vi "Main_RT Feedback.vi"() -> ()   [LabVIEW 2010]
uses:
  <vilib>/Analysis/Matrix/Datatypes/RealMatrix.ctl
  <vilib>/Utility/miscctls.llb/LV3DPointTypeDef.ctl
  <vilib>/Utility/miscctls.llb/LVRectTypeDef.ctl
  <vilib>/picture/3D Picture Control/NI_3D Picture Control.lvlib
  <vilib>/Analysis/Matrix/NI_Matrix.lvlib
panel:
  out "Number of Markers\nfor first BodyDef":i32
  in  "STOP":bool
  out "Unnamed Data":sgl[](array[numeric])
  out "nUnidentifiedMarkers":i32
  out "Unidentified Markers Ptr":u32
  out "Marker Data":sgl[][](array[numeric])
  out "Marker Names\nfor first BodyDef":string[](array[string])
  out "szMarkerNames":u32[](array[numeric])
  out "nMarkers":i32[](array[numeric])
  in  "sBodyDefs":T1
  out "iFrame 2":i32
  in  "Host IP":string="10.1.1.200"
  in  "Local IP":string="10.1.1.150"
  in  "DLL Path":path=path "C:/Program Files (x86)/Motion Analysis/SDK2/Cortex_SDK.dll"
  in  "Write Data to TRC?":bool=TRUE
  out "Arm Refs":T2
  out "3D Picture":refnum<vi>
  in  "Shoulder":bool=TRUE
  out "SceneWindow":refnum<vi>
  # "RealTime Feedback Program for Tracking Shoulder Motion"
  # "Left"
  # "Right"
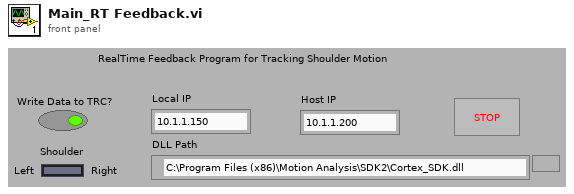
[diagram p1: front panel]
types:
  T1 = cluster{"nBodyDefs":i32, "sBodyDef":cluster{"szName":u32, "nMarkers":i32, "szMarkerNames":u32, "sHierarchy":cluster{"nSegments":i32, "szSegmentNames":u32, "iParents":u32}, "nDofs":i32, "szDefNames":u32}, "nAnalogChannels":i32, "szAnalogChannelNames":u32, "nForcePlates":i32, "AllocatedSpace":u32}
  T2 = cluster{"R Arm":refnum<vi>, "L Arm":refnum<vi>, "R SJC":refnum<vi>, "L EJC":refnum<vi>, "R EJC":refnum<vi>}
  T3 = typedef "NI_Matrix.lvlib/RealMatrix.ctl" = dbl[][]
  T4 = enum16{"Open", "Minimized", "Maximized", "Hidden"}
  T5 = typedef "LV3DPointTypeDef.ctl" = cluster{"X":sgl, "Y":sgl, "Z":sgl}
  T6 = typedef "LVRectTypeDef.ctl" = cluster{"Left":i16, "Top":i16, "Right":i16, "Bottom":i16}
  T7 = cluster{"Shoulder Axis[0]":dbl, "Shoulder Axis[1]":dbl, "Shoulder Axis[2]":dbl}
  T8 = cluster{dbl, "Shoulder Axis":cluster{"Shoulder Axis[0]":dbl, "Shoulder Axis[1]":dbl, "Shoulder Axis[2]":dbl}, dbl, "Shoulder Axis":cluster{"Shoulder Axis[0]":dbl, "Shoulder Axis[1]":dbl, "Shoulder Axis[2]":dbl}, "Humerus Coord Sys":T3, "Shoulder Axis":cluster{"Shoulder Axis[0]":dbl, "Shoulder Axis[1]":dbl, "Shoulder Axis[2]":dbl}}
  T9 = cluster{"szName":u32, "nMarkers":i32, "szMarkerNames":u32, "sHierarchy":cluster{"nSegments":i32, "szSegmentNames":u32, "iParents":u32}, "nDofs":i32, "szDefNames":u32}
  T10 = cluster{"[0]":cluster{"szName":u32, "nMarkers":i32, "szMarkerNames":u32, "sHierarchy":cluster{"nSegments":i32, "szSegmentNames":u32, "iParents":u32}, "nDofs":i32, "szDefNames":u32}, "[1]":cluster{"szName":u32, "nMarkers":i32, "szMarkerNames":u32, "sHierarchy":cluster{"nSegments":i32, "szSegmentNames":u32, "iParents":u32}, "nDofs":i32, "szDefNames":u32}, "[2]":cluster{"szName":u32, "nMarkers":i32, "szMarkerNames":u32, "sHierarchy":cluster{"nSegments":i32, "szSegmentNames":u32, "iParents":u32}, "nDofs":i32, "szDefNames":u32}, "[3]":cluster{"szName":u32, "nMarkers":i32, "szMarkerNames":u32, "sHierarchy":cluster{"nSegments":i32, "szSegmentNames":u32, "iParents":u32}, "nDofs":i32, "szDefNames":u32}, "[4]":cluster{"szName":u32, "nMarkers":i32, "szMarkerNames":u32, "sHierarchy":cluster{"nSegments":i32, "szSegmentNames":u32, "iParents":u32}, "nDofs":i32, "szDefNames":u32}, "[5]":cluster{"szName":u32, "nMarkers":i32, "szMarkerNames":u32, "sHierarchy":cluster{"nSegments":i32, "szSegmentNames":u32, "iParents":u32}, "nDofs":i32, "szDefNames":u32}, "[6]":cluster{"szName":u32, "nMarkers":i32, "szMarkerNames":u32, "sHierarchy":cluster{"nSegments":i32, "szSegmentNames":u32, "iParents":u32}, "nDofs":i32, "szDefNames":u32}, "[7]":cluster{"szName":u32, "nMarkers":i32, "szMarkerNames":u32, "sHierarchy":cluster{"nSegments":i32, "szSegmentNames":u32, "iParents":u32}, "nDofs":i32, "szDefNames":u32}, "[8]":cluster{"szName":u32, "nMarkers":i32, "szMarkerNames":u32, "sHierarchy":cluster{"nSegments":i32, "szSegmentNames":u32, "iParents":u32}, "nDofs":i32, "szDefNames":u32}, "[9]":cluster{"szName":u32, "nMarkers":i32, "szMarkerNames":u32, "sHierarchy":cluster{"nSegments":i32, "szSegmentNames":u32, "iParents":u32}, "nDofs":i32, "szDefNames":u32}, "[10]":cluster{"szName":u32, "nMarkers":i32, "szMarkerNames":u32, "sHierarchy":cluster{"nSegments":i32, "szSegmentNames":u32, "iParents":u32}, "nDofs":i32, "szDefNames":u32}, "[11]":cluster{"szName":u32, "nMarkers":i32, "szMarkerNames":u32, "sHierarchy":cluster{"nSegments":i32, "szSegmentNames":u32, "iParents":u32}, "nDofs":i32, "szDefNames":u32}, "[12]":cluster{"szName":u32, "nMarkers":i32, "szMarkerNames":u32, "sHierarchy":cluster{"nSegments":i32, "szSegmentNames":u32, "iParents":u32}, "nDofs":i32, "szDefNames":u32}, "[13]":cluster{"szName":u32, "nMarkers":i32, "szMarkerNames":u32, "sHierarchy":cluster{"nSegments":i32, "szSegmentNames":u32, "iParents":u32}, "nDofs":i32, "szDefNames":u32}, "[14]":cluster{"szName":u32, "nMarkers":i32, "szMarkerNames":u32, "sHierarchy":cluster{"nSegments":i32, "szSegmentNames":u32, "iParents":u32}, "nDofs":i32, "szDefNames":u32}, "[15]":cluster{"szName":u32, "nMarkers":i32, "szMarkerNames":u32, "sHierarchy":cluster{"nSegments":i32, "szSegmentNames":u32, "iParents":u32}, "nDofs":i32, "szDefNames":u32}, "[16]":cluster{"szName":u32, "nMarkers":i32, "szMarkerNames":u32, "sHierarchy":cluster{"nSegments":i32, "szSegmentNames":u32, "iParents":u32}, "nDofs":i32, "szDefNames":u32}, "[17]":cluster{"szName":u32, "nMarkers":i32, "szMarkerNames":u32, "sHierarchy":cluster{"nSegments":i32, "szSegmentNames":u32, "iParents":u32}, "nDofs":i32, "szDefNames":u32}, "[18]":cluster{"szName":u32, "nMarkers":i32, "szMarkerNames":u32, "sHierarchy":cluster{"nSegments":i32, "szSegmentNames":u32, "iParents":u32}, "nDofs":i32, "szDefNames":u32}, "[19]":cluster{"szName":u32, "nMarkers":i32, "szMarkerNames":u32, "sHierarchy":cluster{"nSegments":i32, "szSegmentNames":u32, "iParents":u32}, "nDofs":i32, "szDefNames":u32}, "[20]":cluster{"szName":u32, "nMarkers":i32, "szMarkerNames":u32, "sHierarchy":cluster{"nSegments":i32, "szSegmentNames":u32, "iParents":u32}, "nDofs":i32, "szDefNames":u32}, "[21]":cluster{"szName":u32, "nMarkers":i32, "szMarkerNames":u32, "sHierarchy":cluster{"nSegments":i32, "szSegmentNames":u32, "iParents":u32}, "nDofs":i32, "szDefNames":u32}, "[22]":cluster{"szName":u32, "nMarkers":i32, "szMarkerNames":u32, "sHierarchy":cluster{"nSegments":i32, "szSegmentNames":u32, "iParents":u32}, "nDofs":i32, "szDefNames":u32}, "[23]":cluster{"szName":u32, "nMarkers":i32, "szMarkerNames":u32, "sHierarchy":cluster{"nSegments":i32, "szSegmentNames":u32, "iParents":u32}, "nDofs":i32, "szDefNames":u32}, "[24]":cluster{"szName":u32, "nMarkers":i32, "szMarkerNames":u32, "sHierarchy":cluster{"nSegments":i32, "szSegmentNames":u32, "iParents":u32}, "nDofs":i32, "szDefNames":u32}, "[25]":cluster{"szName":u32, "nMarkers":i32, "szMarkerNames":u32, "sHierarchy":cluster{"nSegments":i32, "szSegmentNames":u32, "iParents":u32}, "nDofs":i32, "szDefNames":u32}, "[26]":cluster{"szName":u32, "nMarkers":i32, "szMarkerNames":u32, "sHierarchy":cluster{"nSegments":i32, "szSegmentNames":u32, "iParents":u32}, "nDofs":i32, "szDefNames":u32}, "[27]":cluster{"szName":u32, "nMarkers":i32, "szMarkerNames":u32, "sHierarchy":cluster{"nSegments":i32, "szSegmentNames":u32, "iParents":u32}, "nDofs":i32, "szDefNames":u32}, "[28]":cluster{"szName":u32, "nMarkers":i32, "szMarkerNames":u32, "sHierarchy":cluster{"nSegments":i32, "szSegmentNames":u32, "iParents":u32}, "nDofs":i32, "szDefNames":u32}, "[29]":cluster{"szName":u32, "nMarkers":i32, "szMarkerNames":u32, "sHierarchy":cluster{"nSegments":i32, "szSegmentNames":u32, "iParents":u32}, "nDofs":i32, "szDefNames":u32}, "[30]":cluster{"szName":u32, "nMarkers":i32, "szMarkerNames":u32, "sHierarchy":cluster{"nSegments":i32, "szSegmentNames":u32, "iParents":u32}, "nDofs":i32, "szDefNames":u32}, "[31]":cluster{"szName":u32, "nMarkers":i32, "szMarkerNames":u32, "sHierarchy":cluster{"nSegments":i32, "szSegmentNames":u32, "iParents":u32}, "nDofs":i32, "szDefNames":u32}, "[32]":cluster{"szName":u32, "nMarkers":i32, "szMarkerNames":u32, "sHierarchy":cluster{"nSegments":i32, "szSegmentNames":u32, "iParents":u32}, "nDofs":i32, "szDefNames":u32}, "[33]":cluster{"szName":u32, "nMarkers":i32, "szMarkerNames":u32, "sHierarchy":cluster{"nSegments":i32, "szSegmentNames":u32, "iParents":u32}, "nDofs":i32, "szDefNames":u32}, "[34]":cluster{"szName":u32, "nMarkers":i32, "szMarkerNames":u32, "sHierarchy":cluster{"nSegments":i32, "szSegmentNames":u32, "iParents":u32}, "nDofs":i32, "szDefNames":u32}, "[35]":cluster{"szName":u32, "nMarkers":i32, "szMarkerNames":u32, "sHierarchy":cluster{"nSegments":i32, "szSegmentNames":u32, "iParents":u32}, "nDofs":i32, "szDefNames":u32}, "[36]":cluster{"szName":u32, "nMarkers":i32, "szMarkerNames":u32, "sHierarchy":cluster{"nSegments":i32, "szSegmentNames":u32, "iParents":u32}, "nDofs":i32, "szDefNames":u32}, "[37]":cluster{"szName":u32, "nMarkers":i32, "szMarkerNames":u32, "sHierarchy":cluster{"nSegments":i32, "szSegmentNames":u32, "iParents":u32}, "nDofs":i32, "szDefNames":u32}, "[38]":cluster{"szName":u32, "nMarkers":i32, "szMarkerNames":u32, "sHierarchy":cluster{"nSegments":i32, "szSegmentNames":u32, "iParents":u32}, "nDofs":i32, "szDefNames":u32}, "[39]":cluster{"szName":u32, "nMarkers":i32, "szMarkerNames":u32, "sHierarchy":cluster{"nSegments":i32, "szSegmentNames":u32, "iParents":u32}, "nDofs":i32, "szDefNames":u32}, "[40]":cluster{"szName":u32, "nMarkers":i32, "szMarkerNames":u32, "sHierarchy":cluster{"nSegments":i32, "szSegmentNames":u32, "iParents":u32}, "nDofs":i32, "szDefNames":u32}, "[41]":cluster{"szName":u32, "nMarkers":i32, "szMarkerNames":u32, "sHierarchy":cluster{"nSegments":i32, "szSegmentNames":u32, "iParents":u32}, "nDofs":i32, "szDefNames":u32}, "[42]":cluster{"szName":u32, "nMarkers":i32, "szMarkerNames":u32, "sHierarchy":cluster{"nSegments":i32, "szSegmentNames":u32, "iParents":u32}, "nDofs":i32, "szDefNames":u32}, "[43]":cluster{"szName":u32, "nMarkers":i32, "szMarkerNames":u32, "sHierarchy":cluster{"nSegments":i32, "szSegmentNames":u32, "iParents":u32}, "nDofs":i32, "szDefNames":u32}, "[44]":cluster{"szName":u32, "nMarkers":i32, "szMarkerNames":u32, "sHierarchy":cluster{"nSegments":i32, "szSegmentNames":u32, "iParents":u32}, "nDofs":i32, "szDefNames":u32}, "[45]":cluster{"szName":u32, "nMarkers":i32, "szMarkerNames":u32, "sHierarchy":cluster{"nSegments":i32, "szSegmentNames":u32, "iParents":u32}, "nDofs":i32, "szDefNames":u32}, "[46]":cluster{"szName":u32, "nMarkers":i32, "szMarkerNames":u32, "sHierarchy":cluster{"nSegments":i32, "szSegmentNames":u32, "iParents":u32}, "nDofs":i32, "szDefNames":u32}, "[47]":cluster{"szName":u32, "nMarkers":i32, "szMarkerNames":u32, "sHierarchy":cluster{"nSegments":i32, "szSegmentNames":u32, "iParents":u32}, "nDofs":i32, "szDefNames":u32}, "[48]":cluster{"szName":u32, "nMarkers":i32, "szMarkerNames":u32, "sHierarchy":cluster{"nSegments":i32, "szSegmentNames":u32, "iParents":u32}, "nDofs":i32, "szDefNames":u32}, "[49]":cluster{"szName":u32, "nMarkers":i32, "szMarkerNames":u32, "sHierarchy":cluster{"nSegments":i32, "szSegmentNames":u32, "iParents":u32}, "nDofs":i32, "szDefNames":u32}, "[50]":cluster{"szName":u32, "nMarkers":i32, "szMarkerNames":u32, "sHierarchy":cluster{"nSegments":i32, "szSegmentNames":u32, "iParents":u32}, "nDofs":i32, "szDefNames":u32}, "[51]":cluster{"szName":u32, "nMarkers":i32, "szMarkerNames":u32, "sHierarchy":cluster{"nSegments":i32, "szSegmentNames":u32, "iParents":u32}, "nDofs":i32, "szDefNames":u32}, "[52]":cluster{"szName":u32, "nMarkers":i32, "szMarkerNames":u32, "sHierarchy":cluster{"nSegments":i32, "szSegmentNames":u32, "iParents":u32}, "nDofs":i32, "szDefNames":u32}, "[53]":cluster{"szName":u32, "nMarkers":i32, "szMarkerNames":u32, "sHierarchy":cluster{"nSegments":i32, "szSegmentNames":u32, "iParents":u32}, "nDofs":i32, "szDefNames":u32}, "[54]":cluster{"szName":u32, "nMarkers":i32, "szMarkerNames":u32, "sHierarchy":cluster{"nSegments":i32, "szSegmentNames":u32, "iParents":u32}, "nDofs":i32, "szDefNames":u32}, "[55]":cluster{"szName":u32, "nMarkers":i32, "szMarkerNames":u32, "sHierarchy":cluster{"nSegments":i32, "szSegmentNames":u32, "iParents":u32}, "nDofs":i32, "szDefNames":u32}, "[56]":cluster{"szName":u32, "nMarkers":i32, "szMarkerNames":u32, "sHierarchy":cluster{"nSegments":i32, "szSegmentNames":u32, "iParents":u32}, "nDofs":i32, "szDefNames":u32}, "[57]":cluster{"szName":u32, "nMarkers":i32, "szMarkerNames":u32, "sHierarchy":cluster{"nSegments":i32, "szSegmentNames":u32, "iParents":u32}, "nDofs":i32, "szDefNames":u32}, "[58]":cluster{"szName":u32, "nMarkers":i32, "szMarkerNames":u32, "sHierarchy":cluster{"nSegments":i32, "szSegmentNames":u32, "iParents":u32}, "nDofs":i32, "szDefNames":u32}, "[59]":cluster{"szName":u32, "nMarkers":i32, "szMarkerNames":u32, "sHierarchy":cluster{"nSegments":i32, "szSegmentNames":u32, "iParents":u32}, "nDofs":i32, "szDefNames":u32}, "[60]":cluster{"szName":u32, "nMarkers":i32, "szMarkerNames":u32, "sHierarchy":cluster{"nSegments":i32, "szSegmentNames":u32, "iParents":u32}, "nDofs":i32, "szDefNames":u32}, "[61]":cluster{"szName":u32, "nMarkers":i32, "szMarkerNames":u32, "sHierarchy":cluster{"nSegments":i32, "szSegmentNames":u32, "iParents":u32}, "nDofs":i32, "szDefNames":u32}, "[62]":cluster{"szName":u32, "nMarkers":i32, "szMarkerNames":u32, "sHierarchy":cluster{"nSegments":i32, "szSegmentNames":u32, "iParents":u32}, "nDofs":i32, "szDefNames":u32}, "[63]":cluster{"szName":u32, "nMarkers":i32, "szMarkerNames":u32, "sHierarchy":cluster{"nSegments":i32, "szSegmentNames":u32, "iParents":u32}, "nDofs":i32, "szDefNames":u32}, "[64]":cluster{"szName":u32, "nMarkers":i32, "szMarkerNames":u32, "sHierarchy":cluster{"nSegments":i32, "szSegmentNames":u32, "iParents":u32}, "nDofs":i32, "szDefNames":u32}, "[65]":cluster{"szName":u32, "nMarkers":i32, "szMarkerNames":u32, "sHierarchy":cluster{"nSegments":i32, "szSegmentNames":u32, "iParents":u32}, "nDofs":i32, "szDefNames":u32}, "[66]":cluster{"szName":u32, "nMarkers":i32, "szMarkerNames":u32, "sHierarchy":cluster{"nSegments":i32, "szSegmentNames":u32, "iParents":u32}, "nDofs":i32, "szDefNames":u32}, "[67]":cluster{"szName":u32, "nMarkers":i32, "szMarkerNames":u32, "sHierarchy":cluster{"nSegments":i32, "szSegmentNames":u32, "iParents":u32}, "nDofs":i32, "szDefNames":u32}, "[68]":cluster{"szName":u32, "nMarkers":i32, "szMarkerNames":u32, "sHierarchy":cluster{"nSegments":i32, "szSegmentNames":u32, "iParents":u32}, "nDofs":i32, "szDefNames":u32}, "[69]":cluster{"szName":u32, "nMarkers":i32, "szMarkerNames":u32, "sHierarchy":cluster{"nSegments":i32, "szSegmentNames":u32, "iParents":u32}, "nDofs":i32, "szDefNames":u32}, "[70]":cluster{"szName":u32, "nMarkers":i32, "szMarkerNames":u32, "sHierarchy":cluster{"nSegments":i32, "szSegmentNames":u32, "iParents":u32}, "nDofs":i32, "szDefNames":u32}, "[71]":cluster{"szName":u32, "nMarkers":i32, "szMarkerNames":u32, "sHierarchy":cluster{"nSegments":i32, "szSegmentNames":u32, "iParents":u32}, "nDofs":i32, "szDefNames":u32}, "[72]":cluster{"szName":u32, "nMarkers":i32, "szMarkerNames":u32, "sHierarchy":cluster{"nSegments":i32, "szSegmentNames":u32, "iParents":u32}, "nDofs":i32, "szDefNames":u32}, "[73]":cluster{"szName":u32, "nMarkers":i32, "szMarkerNames":u32, "sHierarchy":cluster{"nSegments":i32, "szSegmentNames":u32, "iParents":u32}, "nDofs":i32, "szDefNames":u32}, "[74]":cluster{"szName":u32, "nMarkers":i32, "szMarkerNames":u32, "sHierarchy":cluster{"nSegments":i32, "szSegmentNames":u32, "iParents":u32}, "nDofs":i32, "szDefNames":u32}, "[75]":cluster{"szName":u32, "nMarkers":i32, "szMarkerNames":u32, "sHierarchy":cluster{"nSegments":i32, "szSegmentNames":u32, "iParents":u32}, "nDofs":i32, "szDefNames":u32}, "[76]":cluster{"szName":u32, "nMarkers":i32, "szMarkerNames":u32, "sHierarchy":cluster{"nSegments":i32, "szSegmentNames":u32, "iParents":u32}, "nDofs":i32, "szDefNames":u32}, "[77]":cluster{"szName":u32, "nMarkers":i32, "szMarkerNames":u32, "sHierarchy":cluster{"nSegments":i32, "szSegmentNames":u32, "iParents":u32}, "nDofs":i32, "szDefNames":u32}, "[78]":cluster{"szName":u32, "nMarkers":i32, "szMarkerNames":u32, "sHierarchy":cluster{"nSegments":i32, "szSegmentNames":u32, "iParents":u32}, "nDofs":i32, "szDefNames":u32}, "[79]":cluster{"szName":u32, "nMarkers":i32, "szMarkerNames":u32, "sHierarchy":cluster{"nSegments":i32, "szSegmentNames":u32, "iParents":u32}, "nDofs":i32, "szDefNames":u32}, "[80]":cluster{"szName":u32, "nMarkers":i32, "szMarkerNames":u32, "sHierarchy":cluster{"nSegments":i32, "szSegmentNames":u32, "iParents":u32}, "nDofs":i32, "szDefNames":u32}, "[81]":cluster{"szName":u32, "nMarkers":i32, "szMarkerNames":u32, "sHierarchy":cluster{"nSegments":i32, "szSegmentNames":u32, "iParents":u32}, "nDofs":i32, "szDefNames":u32}, "[82]":cluster{"szName":u32, "nMarkers":i32, "szMarkerNames":u32, "sHierarchy":cluster{"nSegments":i32, "szSegmentNames":u32, "iParents":u32}, "nDofs":i32, "szDefNames":u32}, "[83]":cluster{"szName":u32, "nMarkers":i32, "szMarkerNames":u32, "sHierarchy":cluster{"nSegments":i32, "szSegmentNames":u32, "iParents":u32}, "nDofs":i32, "szDefNames":u32}, "[84]":cluster{"szName":u32, "nMarkers":i32, "szMarkerNames":u32, "sHierarchy":cluster{"nSegments":i32, "szSegmentNames":u32, "iParents":u32}, "nDofs":i32, "szDefNames":u32}, "[85]":cluster{"szName":u32, "nMarkers":i32, "szMarkerNames":u32, "sHierarchy":cluster{"nSegments":i32, "szSegmentNames":u32, "iParents":u32}, "nDofs":i32, "szDefNames":u32}, "[86]":cluster{"szName":u32, "nMarkers":i32, "szMarkerNames":u32, "sHierarchy":cluster{"nSegments":i32, "szSegmentNames":u32, "iParents":u32}, "nDofs":i32, "szDefNames":u32}, "[87]":cluster{"szName":u32, "nMarkers":i32, "szMarkerNames":u32, "sHierarchy":cluster{"nSegments":i32, "szSegmentNames":u32, "iParents":u32}, "nDofs":i32, "szDefNames":u32}, "[88]":cluster{"szName":u32, "nMarkers":i32, "szMarkerNames":u32, "sHierarchy":cluster{"nSegments":i32, "szSegmentNames":u32, "iParents":u32}, "nDofs":i32, "szDefNames":u32}, "[89]":cluster{"szName":u32, "nMarkers":i32, "szMarkerNames":u32, "sHierarchy":cluster{"nSegments":i32, "szSegmentNames":u32, "iParents":u32}, "nDofs":i32, "szDefNames":u32}, "[90]":cluster{"szName":u32, "nMarkers":i32, "szMarkerNames":u32, "sHierarchy":cluster{"nSegments":i32, "szSegmentNames":u32, "iParents":u32}, "nDofs":i32, "szDefNames":u32}, "[91]":cluster{"szName":u32, "nMarkers":i32, "szMarkerNames":u32, "sHierarchy":cluster{"nSegments":i32, "szSegmentNames":u32, "iParents":u32}, "nDofs":i32, "szDefNames":u32}, "[92]":cluster{"szName":u32, "nMarkers":i32, "szMarkerNames":u32, "sHierarchy":cluster{"nSegments":i32, "szSegmentNames":u32, "iParents":u32}, "nDofs":i32, "szDefNames":u32}, "[93]":cluster{"szName":u32, "nMarkers":i32, "szMarkerNames":u32, "sHierarchy":cluster{"nSegments":i32, "szSegmentNames":u32, "iParents":u32}, "nDofs":i32, "szDefNames":u32}, "[94]":cluster{"szName":u32, "nMarkers":i32, "szMarkerNames":u32, "sHierarchy":cluster{"nSegments":i32, "szSegmentNames":u32, "iParents":u32}, "nDofs":i32, "szDefNames":u32}, "[95]":cluster{"szName":u32, "nMarkers":i32, "szMarkerNames":u32, "sHierarchy":cluster{"nSegments":i32, "szSegmentNames":u32, "iParents":u32}, "nDofs":i32, "szDefNames":u32}, "[96]":cluster{"szName":u32, "nMarkers":i32, "szMarkerNames":u32, "sHierarchy":cluster{"nSegments":i32, "szSegmentNames":u32, "iParents":u32}, "nDofs":i32, "szDefNames":u32}, "[97]":cluster{"szName":u32, "nMarkers":i32, "szMarkerNames":u32, "sHierarchy":cluster{"nSegments":i32, "szSegmentNames":u32, "iParents":u32}, "nDofs":i32, "szDefNames":u32}, "[98]":cluster{"szName":u32, "nMarkers":i32, "szMarkerNames":u32, "sHierarchy":cluster{"nSegments":i32, "szSegmentNames":u32, "iParents":u32}, "nDofs":i32, "szDefNames":u32}, "[99]":cluster{"szName":u32, "nMarkers":i32, "szMarkerNames":u32, "sHierarchy":cluster{"nSegments":i32, "szSegmentNames":u32, "iParents":u32}, "nDofs":i32, "szDefNames":u32}}
  T11 = cluster{"nBodyDefs":i32, cluster{"[0]":cluster{"szName":u32, "nMarkers":i32, "szMarkerNames":u32, "sHierarchy":cluster{"nSegments":i32, "szSegmentNames":u32, "iParents":u32}, "nDofs":i32, "szDefNames":u32}, "[1]":cluster{"szName":u32, "nMarkers":i32, "szMarkerNames":u32, "sHierarchy":cluster{"nSegments":i32, "szSegmentNames":u32, "iParents":u32}, "nDofs":i32, "szDefNames":u32}, "[2]":cluster{"szName":u32, "nMarkers":i32, "szMarkerNames":u32, "sHierarchy":cluster{"nSegments":i32, "szSegmentNames":u32, "iParents":u32}, "nDofs":i32, "szDefNames":u32}, "[3]":cluster{"szName":u32, "nMarkers":i32, "szMarkerNames":u32, "sHierarchy":cluster{"nSegments":i32, "szSegmentNames":u32, "iParents":u32}, "nDofs":i32, "szDefNames":u32}, "[4]":cluster{"szName":u32, "nMarkers":i32, "szMarkerNames":u32, "sHierarchy":cluster{"nSegments":i32, "szSegmentNames":u32, "iParents":u32}, "nDofs":i32, "szDefNames":u32}, "[5]":cluster{"szName":u32, "nMarkers":i32, "szMarkerNames":u32, "sHierarchy":cluster{"nSegments":i32, "szSegmentNames":u32, "iParents":u32}, "nDofs":i32, "szDefNames":u32}, "[6]":cluster{"szName":u32, "nMarkers":i32, "szMarkerNames":u32, "sHierarchy":cluster{"nSegments":i32, "szSegmentNames":u32, "iParents":u32}, "nDofs":i32, "szDefNames":u32}, "[7]":cluster{"szName":u32, "nMarkers":i32, "szMarkerNames":u32, "sHierarchy":cluster{"nSegments":i32, "szSegmentNames":u32, "iParents":u32}, "nDofs":i32, "szDefNames":u32}, "[8]":cluster{"szName":u32, "nMarkers":i32, "szMarkerNames":u32, "sHierarchy":cluster{"nSegments":i32, "szSegmentNames":u32, "iParents":u32}, "nDofs":i32, "szDefNames":u32}, "[9]":cluster{"szName":u32, "nMarkers":i32, "szMarkerNames":u32, "sHierarchy":cluster{"nSegments":i32, "szSegmentNames":u32, "iParents":u32}, "nDofs":i32, "szDefNames":u32}, "[10]":cluster{"szName":u32, "nMarkers":i32, "szMarkerNames":u32, "sHierarchy":cluster{"nSegments":i32, "szSegmentNames":u32, "iParents":u32}, "nDofs":i32, "szDefNames":u32}, "[11]":cluster{"szName":u32, "nMarkers":i32, "szMarkerNames":u32, "sHierarchy":cluster{"nSegments":i32, "szSegmentNames":u32, "iParents":u32}, "nDofs":i32, "szDefNames":u32}, "[12]":cluster{"szName":u32, "nMarkers":i32, "szMarkerNames":u32, "sHierarchy":cluster{"nSegments":i32, "szSegmentNames":u32, "iParents":u32}, "nDofs":i32, "szDefNames":u32}, "[13]":cluster{"szName":u32, "nMarkers":i32, "szMarkerNames":u32, "sHierarchy":cluster{"nSegments":i32, "szSegmentNames":u32, "iParents":u32}, "nDofs":i32, "szDefNames":u32}, "[14]":cluster{"szName":u32, "nMarkers":i32, "szMarkerNames":u32, "sHierarchy":cluster{"nSegments":i32, "szSegmentNames":u32, "iParents":u32}, "nDofs":i32, "szDefNames":u32}, "[15]":cluster{"szName":u32, "nMarkers":i32, "szMarkerNames":u32, "sHierarchy":cluster{"nSegments":i32, "szSegmentNames":u32, "iParents":u32}, "nDofs":i32, "szDefNames":u32}, "[16]":cluster{"szName":u32, "nMarkers":i32, "szMarkerNames":u32, "sHierarchy":cluster{"nSegments":i32, "szSegmentNames":u32, "iParents":u32}, "nDofs":i32, "szDefNames":u32}, "[17]":cluster{"szName":u32, "nMarkers":i32, "szMarkerNames":u32, "sHierarchy":cluster{"nSegments":i32, "szSegmentNames":u32, "iParents":u32}, "nDofs":i32, "szDefNames":u32}, "[18]":cluster{"szName":u32, "nMarkers":i32, "szMarkerNames":u32, "sHierarchy":cluster{"nSegments":i32, "szSegmentNames":u32, "iParents":u32}, "nDofs":i32, "szDefNames":u32}, "[19]":cluster{"szName":u32, "nMarkers":i32, "szMarkerNames":u32, "sHierarchy":cluster{"nSegments":i32, "szSegmentNames":u32, "iParents":u32}, "nDofs":i32, "szDefNames":u32}, "[20]":cluster{"szName":u32, "nMarkers":i32, "szMarkerNames":u32, "sHierarchy":cluster{"nSegments":i32, "szSegmentNames":u32, "iParents":u32}, "nDofs":i32, "szDefNames":u32}, "[21]":cluster{"szName":u32, "nMarkers":i32, "szMarkerNames":u32, "sHierarchy":cluster{"nSegments":i32, "szSegmentNames":u32, "iParents":u32}, "nDofs":i32, "szDefNames":u32}, "[22]":cluster{"szName":u32, "nMarkers":i32, "szMarkerNames":u32, "sHierarchy":cluster{"nSegments":i32, "szSegmentNames":u32, "iParents":u32}, "nDofs":i32, "szDefNames":u32}, "[23]":cluster{"szName":u32, "nMarkers":i32, "szMarkerNames":u32, "sHierarchy":cluster{"nSegments":i32, "szSegmentNames":u32, "iParents":u32}, "nDofs":i32, "szDefNames":u32}, "[24]":cluster{"szName":u32, "nMarkers":i32, "szMarkerNames":u32, "sHierarchy":cluster{"nSegments":i32, "szSegmentNames":u32, "iParents":u32}, "nDofs":i32, "szDefNames":u32}, "[25]":cluster{"szName":u32, "nMarkers":i32, "szMarkerNames":u32, "sHierarchy":cluster{"nSegments":i32, "szSegmentNames":u32, "iParents":u32}, "nDofs":i32, "szDefNames":u32}, "[26]":cluster{"szName":u32, "nMarkers":i32, "szMarkerNames":u32, "sHierarchy":cluster{"nSegments":i32, "szSegmentNames":u32, "iParents":u32}, "nDofs":i32, "szDefNames":u32}, "[27]":cluster{"szName":u32, "nMarkers":i32, "szMarkerNames":u32, "sHierarchy":cluster{"nSegments":i32, "szSegmentNames":u32, "iParents":u32}, "nDofs":i32, "szDefNames":u32}, "[28]":cluster{"szName":u32, "nMarkers":i32, "szMarkerNames":u32, "sHierarchy":cluster{"nSegments":i32, "szSegmentNames":u32, "iParents":u32}, "nDofs":i32, "szDefNames":u32}, "[29]":cluster{"szName":u32, "nMarkers":i32, "szMarkerNames":u32, "sHierarchy":cluster{"nSegments":i32, "szSegmentNames":u32, "iParents":u32}, "nDofs":i32, "szDefNames":u32}, "[30]":cluster{"szName":u32, "nMarkers":i32, "szMarkerNames":u32, "sHierarchy":cluster{"nSegments":i32, "szSegmentNames":u32, "iParents":u32}, "nDofs":i32, "szDefNames":u32}, "[31]":cluster{"szName":u32, "nMarkers":i32, "szMarkerNames":u32, "sHierarchy":cluster{"nSegments":i32, "szSegmentNames":u32, "iParents":u32}, "nDofs":i32, "szDefNames":u32}, "[32]":cluster{"szName":u32, "nMarkers":i32, "szMarkerNames":u32, "sHierarchy":cluster{"nSegments":i32, "szSegmentNames":u32, "iParents":u32}, "nDofs":i32, "szDefNames":u32}, "[33]":cluster{"szName":u32, "nMarkers":i32, "szMarkerNames":u32, "sHierarchy":cluster{"nSegments":i32, "szSegmentNames":u32, "iParents":u32}, "nDofs":i32, "szDefNames":u32}, "[34]":cluster{"szName":u32, "nMarkers":i32, "szMarkerNames":u32, "sHierarchy":cluster{"nSegments":i32, "szSegmentNames":u32, "iParents":u32}, "nDofs":i32, "szDefNames":u32}, "[35]":cluster{"szName":u32, "nMarkers":i32, "szMarkerNames":u32, "sHierarchy":cluster{"nSegments":i32, "szSegmentNames":u32, "iParents":u32}, "nDofs":i32, "szDefNames":u32}, "[36]":cluster{"szName":u32, "nMarkers":i32, "szMarkerNames":u32, "sHierarchy":cluster{"nSegments":i32, "szSegmentNames":u32, "iParents":u32}, "nDofs":i32, "szDefNames":u32}, "[37]":cluster{"szName":u32, "nMarkers":i32, "szMarkerNames":u32, "sHierarchy":cluster{"nSegments":i32, "szSegmentNames":u32, "iParents":u32}, "nDofs":i32, "szDefNames":u32}, "[38]":cluster{"szName":u32, "nMarkers":i32, "szMarkerNames":u32, "sHierarchy":cluster{"nSegments":i32, "szSegmentNames":u32, "iParents":u32}, "nDofs":i32, "szDefNames":u32}, "[39]":cluster{"szName":u32, "nMarkers":i32, "szMarkerNames":u32, "sHierarchy":cluster{"nSegments":i32, "szSegmentNames":u32, "iParents":u32}, "nDofs":i32, "szDefNames":u32}, "[40]":cluster{"szName":u32, "nMarkers":i32, "szMarkerNames":u32, "sHierarchy":cluster{"nSegments":i32, "szSegmentNames":u32, "iParents":u32}, "nDofs":i32, "szDefNames":u32}, "[41]":cluster{"szName":u32, "nMarkers":i32, "szMarkerNames":u32, "sHierarchy":cluster{"nSegments":i32, "szSegmentNames":u32, "iParents":u32}, "nDofs":i32, "szDefNames":u32}, "[42]":cluster{"szName":u32, "nMarkers":i32, "szMarkerNames":u32, "sHierarchy":cluster{"nSegments":i32, "szSegmentNames":u32, "iParents":u32}, "nDofs":i32, "szDefNames":u32}, "[43]":cluster{"szName":u32, "nMarkers":i32, "szMarkerNames":u32, "sHierarchy":cluster{"nSegments":i32, "szSegmentNames":u32, "iParents":u32}, "nDofs":i32, "szDefNames":u32}, "[44]":cluster{"szName":u32, "nMarkers":i32, "szMarkerNames":u32, "sHierarchy":cluster{"nSegments":i32, "szSegmentNames":u32, "iParents":u32}, "nDofs":i32, "szDefNames":u32}, "[45]":cluster{"szName":u32, "nMarkers":i32, "szMarkerNames":u32, "sHierarchy":cluster{"nSegments":i32, "szSegmentNames":u32, "iParents":u32}, "nDofs":i32, "szDefNames":u32}, "[46]":cluster{"szName":u32, "nMarkers":i32, "szMarkerNames":u32, "sHierarchy":cluster{"nSegments":i32, "szSegmentNames":u32, "iParents":u32}, "nDofs":i32, "szDefNames":u32}, "[47]":cluster{"szName":u32, "nMarkers":i32, "szMarkerNames":u32, "sHierarchy":cluster{"nSegments":i32, "szSegmentNames":u32, "iParents":u32}, "nDofs":i32, "szDefNames":u32}, "[48]":cluster{"szName":u32, "nMarkers":i32, "szMarkerNames":u32, "sHierarchy":cluster{"nSegments":i32, "szSegmentNames":u32, "iParents":u32}, "nDofs":i32, "szDefNames":u32}, "[49]":cluster{"szName":u32, "nMarkers":i32, "szMarkerNames":u32, "sHierarchy":cluster{"nSegments":i32, "szSegmentNames":u32, "iParents":u32}, "nDofs":i32, "szDefNames":u32}, "[50]":cluster{"szName":u32, "nMarkers":i32, "szMarkerNames":u32, "sHierarchy":cluster{"nSegments":i32, "szSegmentNames":u32, "iParents":u32}, "nDofs":i32, "szDefNames":u32}, "[51]":cluster{"szName":u32, "nMarkers":i32, "szMarkerNames":u32, "sHierarchy":cluster{"nSegments":i32, "szSegmentNames":u32, "iParents":u32}, "nDofs":i32, "szDefNames":u32}, "[52]":cluster{"szName":u32, "nMarkers":i32, "szMarkerNames":u32, "sHierarchy":cluster{"nSegments":i32, "szSegmentNames":u32, "iParents":u32}, "nDofs":i32, "szDefNames":u32}, "[53]":cluster{"szName":u32, "nMarkers":i32, "szMarkerNames":u32, "sHierarchy":cluster{"nSegments":i32, "szSegmentNames":u32, "iParents":u32}, "nDofs":i32, "szDefNames":u32}, "[54]":cluster{"szName":u32, "nMarkers":i32, "szMarkerNames":u32, "sHierarchy":cluster{"nSegments":i32, "szSegmentNames":u32, "iParents":u32}, "nDofs":i32, "szDefNames":u32}, "[55]":cluster{"szName":u32, "nMarkers":i32, "szMarkerNames":u32, "sHierarchy":cluster{"nSegments":i32, "szSegmentNames":u32, "iParents":u32}, "nDofs":i32, "szDefNames":u32}, "[56]":cluster{"szName":u32, "nMarkers":i32, "szMarkerNames":u32, "sHierarchy":cluster{"nSegments":i32, "szSegmentNames":u32, "iParents":u32}, "nDofs":i32, "szDefNames":u32}, "[57]":cluster{"szName":u32, "nMarkers":i32, "szMarkerNames":u32, "sHierarchy":cluster{"nSegments":i32, "szSegmentNames":u32, "iParents":u32}, "nDofs":i32, "szDefNames":u32}, "[58]":cluster{"szName":u32, "nMarkers":i32, "szMarkerNames":u32, "sHierarchy":cluster{"nSegments":i32, "szSegmentNames":u32, "iParents":u32}, "nDofs":i32, "szDefNames":u32}, "[59]":cluster{"szName":u32, "nMarkers":i32, "szMarkerNames":u32, "sHierarchy":cluster{"nSegments":i32, "szSegmentNames":u32, "iParents":u32}, "nDofs":i32, "szDefNames":u32}, "[60]":cluster{"szName":u32, "nMarkers":i32, "szMarkerNames":u32, "sHierarchy":cluster{"nSegments":i32, "szSegmentNames":u32, "iParents":u32}, "nDofs":i32, "szDefNames":u32}, "[61]":cluster{"szName":u32, "nMarkers":i32, "szMarkerNames":u32, "sHierarchy":cluster{"nSegments":i32, "szSegmentNames":u32, "iParents":u32}, "nDofs":i32, "szDefNames":u32}, "[62]":cluster{"szName":u32, "nMarkers":i32, "szMarkerNames":u32, "sHierarchy":cluster{"nSegments":i32, "szSegmentNames":u32, "iParents":u32}, "nDofs":i32, "szDefNames":u32}, "[63]":cluster{"szName":u32, "nMarkers":i32, "szMarkerNames":u32, "sHierarchy":cluster{"nSegments":i32, "szSegmentNames":u32, "iParents":u32}, "nDofs":i32, "szDefNames":u32}, "[64]":cluster{"szName":u32, "nMarkers":i32, "szMarkerNames":u32, "sHierarchy":cluster{"nSegments":i32, "szSegmentNames":u32, "iParents":u32}, "nDofs":i32, "szDefNames":u32}, "[65]":cluster{"szName":u32, "nMarkers":i32, "szMarkerNames":u32, "sHierarchy":cluster{"nSegments":i32, "szSegmentNames":u32, "iParents":u32}, "nDofs":i32, "szDefNames":u32}, "[66]":cluster{"szName":u32, "nMarkers":i32, "szMarkerNames":u32, "sHierarchy":cluster{"nSegments":i32, "szSegmentNames":u32, "iParents":u32}, "nDofs":i32, "szDefNames":u32}, "[67]":cluster{"szName":u32, "nMarkers":i32, "szMarkerNames":u32, "sHierarchy":cluster{"nSegments":i32, "szSegmentNames":u32, "iParents":u32}, "nDofs":i32, "szDefNames":u32}, "[68]":cluster{"szName":u32, "nMarkers":i32, "szMarkerNames":u32, "sHierarchy":cluster{"nSegments":i32, "szSegmentNames":u32, "iParents":u32}, "nDofs":i32, "szDefNames":u32}, "[69]":cluster{"szName":u32, "nMarkers":i32, "szMarkerNames":u32, "sHierarchy":cluster{"nSegments":i32, "szSegmentNames":u32, "iParents":u32}, "nDofs":i32, "szDefNames":u32}, "[70]":cluster{"szName":u32, "nMarkers":i32, "szMarkerNames":u32, "sHierarchy":cluster{"nSegments":i32, "szSegmentNames":u32, "iParents":u32}, "nDofs":i32, "szDefNames":u32}, "[71]":cluster{"szName":u32, "nMarkers":i32, "szMarkerNames":u32, "sHierarchy":cluster{"nSegments":i32, "szSegmentNames":u32, "iParents":u32}, "nDofs":i32, "szDefNames":u32}, "[72]":cluster{"szName":u32, "nMarkers":i32, "szMarkerNames":u32, "sHierarchy":cluster{"nSegments":i32, "szSegmentNames":u32, "iParents":u32}, "nDofs":i32, "szDefNames":u32}, "[73]":cluster{"szName":u32, "nMarkers":i32, "szMarkerNames":u32, "sHierarchy":cluster{"nSegments":i32, "szSegmentNames":u32, "iParents":u32}, "nDofs":i32, "szDefNames":u32}, "[74]":cluster{"szName":u32, "nMarkers":i32, "szMarkerNames":u32, "sHierarchy":cluster{"nSegments":i32, "szSegmentNames":u32, "iParents":u32}, "nDofs":i32, "szDefNames":u32}, "[75]":cluster{"szName":u32, "nMarkers":i32, "szMarkerNames":u32, "sHierarchy":cluster{"nSegments":i32, "szSegmentNames":u32, "iParents":u32}, "nDofs":i32, "szDefNames":u32}, "[76]":cluster{"szName":u32, "nMarkers":i32, "szMarkerNames":u32, "sHierarchy":cluster{"nSegments":i32, "szSegmentNames":u32, "iParents":u32}, "nDofs":i32, "szDefNames":u32}, "[77]":cluster{"szName":u32, "nMarkers":i32, "szMarkerNames":u32, "sHierarchy":cluster{"nSegments":i32, "szSegmentNames":u32, "iParents":u32}, "nDofs":i32, "szDefNames":u32}, "[78]":cluster{"szName":u32, "nMarkers":i32, "szMarkerNames":u32, "sHierarchy":cluster{"nSegments":i32, "szSegmentNames":u32, "iParents":u32}, "nDofs":i32, "szDefNames":u32}, "[79]":cluster{"szName":u32, "nMarkers":i32, "szMarkerNames":u32, "sHierarchy":cluster{"nSegments":i32, "szSegmentNames":u32, "iParents":u32}, "nDofs":i32, "szDefNames":u32}, "[80]":cluster{"szName":u32, "nMarkers":i32, "szMarkerNames":u32, "sHierarchy":cluster{"nSegments":i32, "szSegmentNames":u32, "iParents":u32}, "nDofs":i32, "szDefNames":u32}, "[81]":cluster{"szName":u32, "nMarkers":i32, "szMarkerNames":u32, "sHierarchy":cluster{"nSegments":i32, "szSegmentNames":u32, "iParents":u32}, "nDofs":i32, "szDefNames":u32}, "[82]":cluster{"szName":u32, "nMarkers":i32, "szMarkerNames":u32, "sHierarchy":cluster{"nSegments":i32, "szSegmentNames":u32, "iParents":u32}, "nDofs":i32, "szDefNames":u32}, "[83]":cluster{"szName":u32, "nMarkers":i32, "szMarkerNames":u32, "sHierarchy":cluster{"nSegments":i32, "szSegmentNames":u32, "iParents":u32}, "nDofs":i32, "szDefNames":u32}, "[84]":cluster{"szName":u32, "nMarkers":i32, "szMarkerNames":u32, "sHierarchy":cluster{"nSegments":i32, "szSegmentNames":u32, "iParents":u32}, "nDofs":i32, "szDefNames":u32}, "[85]":cluster{"szName":u32, "nMarkers":i32, "szMarkerNames":u32, "sHierarchy":cluster{"nSegments":i32, "szSegmentNames":u32, "iParents":u32}, "nDofs":i32, "szDefNames":u32}, "[86]":cluster{"szName":u32, "nMarkers":i32, "szMarkerNames":u32, "sHierarchy":cluster{"nSegments":i32, "szSegmentNames":u32, "iParents":u32}, "nDofs":i32, "szDefNames":u32}, "[87]":cluster{"szName":u32, "nMarkers":i32, "szMarkerNames":u32, "sHierarchy":cluster{"nSegments":i32, "szSegmentNames":u32, "iParents":u32}, "nDofs":i32, "szDefNames":u32}, "[88]":cluster{"szName":u32, "nMarkers":i32, "szMarkerNames":u32, "sHierarchy":cluster{"nSegments":i32, "szSegmentNames":u32, "iParents":u32}, "nDofs":i32, "szDefNames":u32}, "[89]":cluster{"szName":u32, "nMarkers":i32, "szMarkerNames":u32, "sHierarchy":cluster{"nSegments":i32, "szSegmentNames":u32, "iParents":u32}, "nDofs":i32, "szDefNames":u32}, "[90]":cluster{"szName":u32, "nMarkers":i32, "szMarkerNames":u32, "sHierarchy":cluster{"nSegments":i32, "szSegmentNames":u32, "iParents":u32}, "nDofs":i32, "szDefNames":u32}, "[91]":cluster{"szName":u32, "nMarkers":i32, "szMarkerNames":u32, "sHierarchy":cluster{"nSegments":i32, "szSegmentNames":u32, "iParents":u32}, "nDofs":i32, "szDefNames":u32}, "[92]":cluster{"szName":u32, "nMarkers":i32, "szMarkerNames":u32, "sHierarchy":cluster{"nSegments":i32, "szSegmentNames":u32, "iParents":u32}, "nDofs":i32, "szDefNames":u32}, "[93]":cluster{"szName":u32, "nMarkers":i32, "szMarkerNames":u32, "sHierarchy":cluster{"nSegments":i32, "szSegmentNames":u32, "iParents":u32}, "nDofs":i32, "szDefNames":u32}, "[94]":cluster{"szName":u32, "nMarkers":i32, "szMarkerNames":u32, "sHierarchy":cluster{"nSegments":i32, "szSegmentNames":u32, "iParents":u32}, "nDofs":i32, "szDefNames":u32}, "[95]":cluster{"szName":u32, "nMarkers":i32, "szMarkerNames":u32, "sHierarchy":cluster{"nSegments":i32, "szSegmentNames":u32, "iParents":u32}, "nDofs":i32, "szDefNames":u32}, "[96]":cluster{"szName":u32, "nMarkers":i32, "szMarkerNames":u32, "sHierarchy":cluster{"nSegments":i32, "szSegmentNames":u32, "iParents":u32}, "nDofs":i32, "szDefNames":u32}, "[97]":cluster{"szName":u32, "nMarkers":i32, "szMarkerNames":u32, "sHierarchy":cluster{"nSegments":i32, "szSegmentNames":u32, "iParents":u32}, "nDofs":i32, "szDefNames":u32}, "[98]":cluster{"szName":u32, "nMarkers":i32, "szMarkerNames":u32, "sHierarchy":cluster{"nSegments":i32, "szSegmentNames":u32, "iParents":u32}, "nDofs":i32, "szDefNames":u32}, "[99]":cluster{"szName":u32, "nMarkers":i32, "szMarkerNames":u32, "sHierarchy":cluster{"nSegments":i32, "szSegmentNames":u32, "iParents":u32}, "nDofs":i32, "szDefNames":u32}}, "nAnalogChannels":i32, "szAnalogChannelNames":u32, "nForcePlates":i32, "AllocatedSpace":u32}
  T12 = cluster{"szName":u32, "nMarkers":i32, "szMarkerNames":u32, "sHierarchy":cluster{"nSegments":i32, "szSegmentNames":u32, "iParents":u32}, "nDofs":i32, "szDefNames":u32}[]
  T13 = cluster{"Theta":dbl, "Vector":cluster{"Vector[0]":ext, "Vector[1]":ext, "Vector[2]":ext}, "Theta":dbl, "Vector":cluster{"Vector[0]":ext, "Vector[1]":ext, "Vector[2]":ext}, "Humerus rel Trunk":T3}
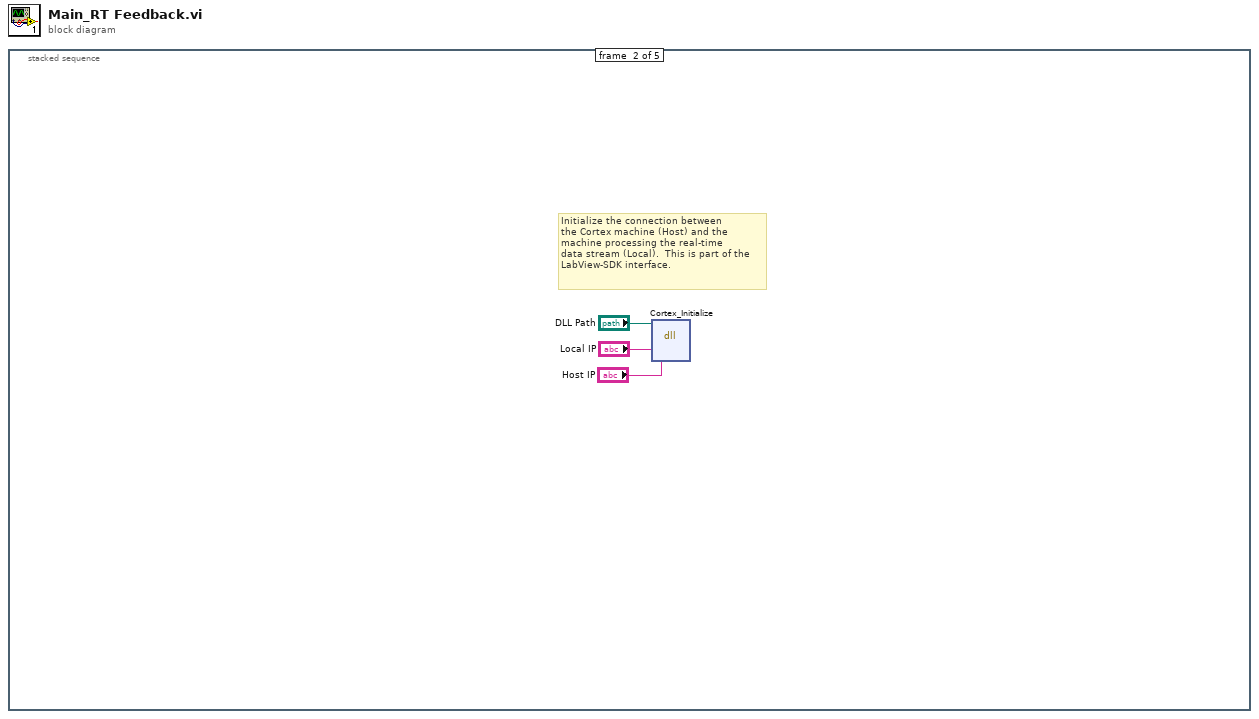
[diagram p0: block diagram]
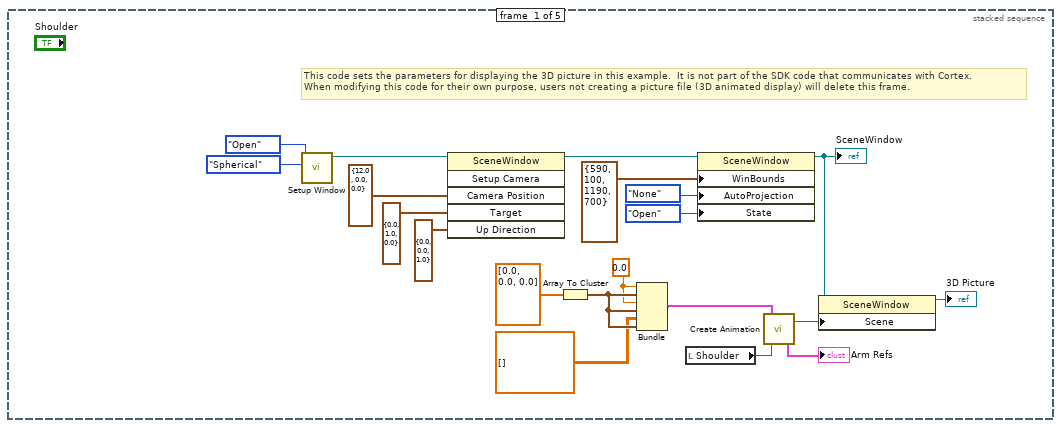
[diagram p2: hidden frame]
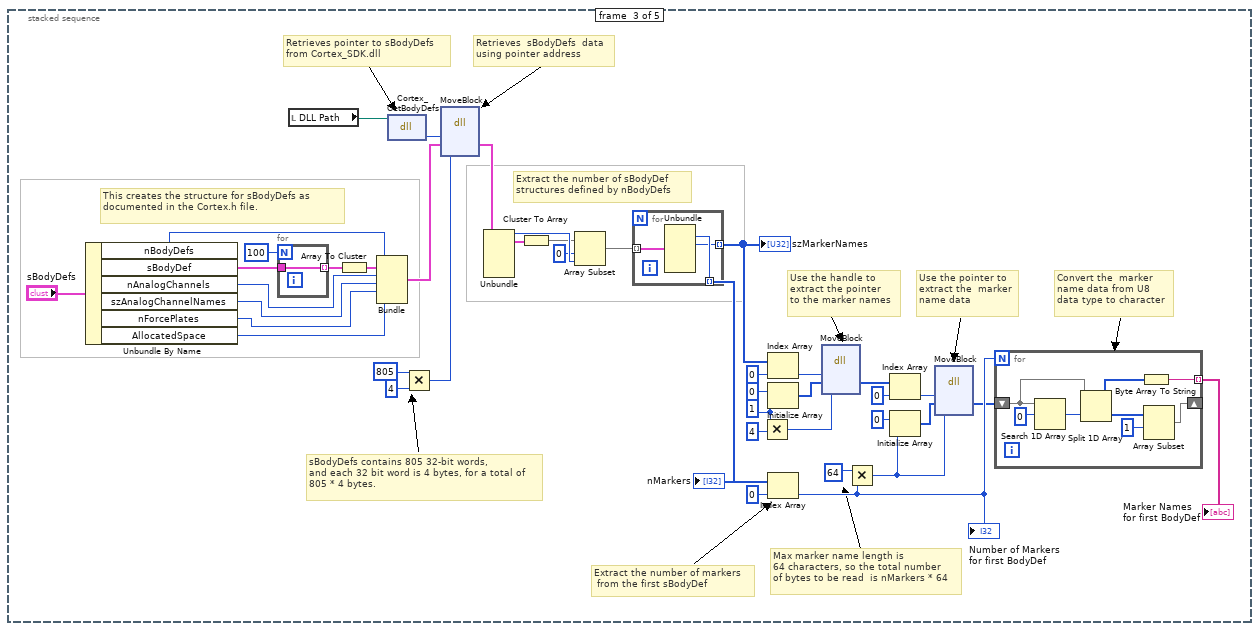
[diagram p3: hidden frame]
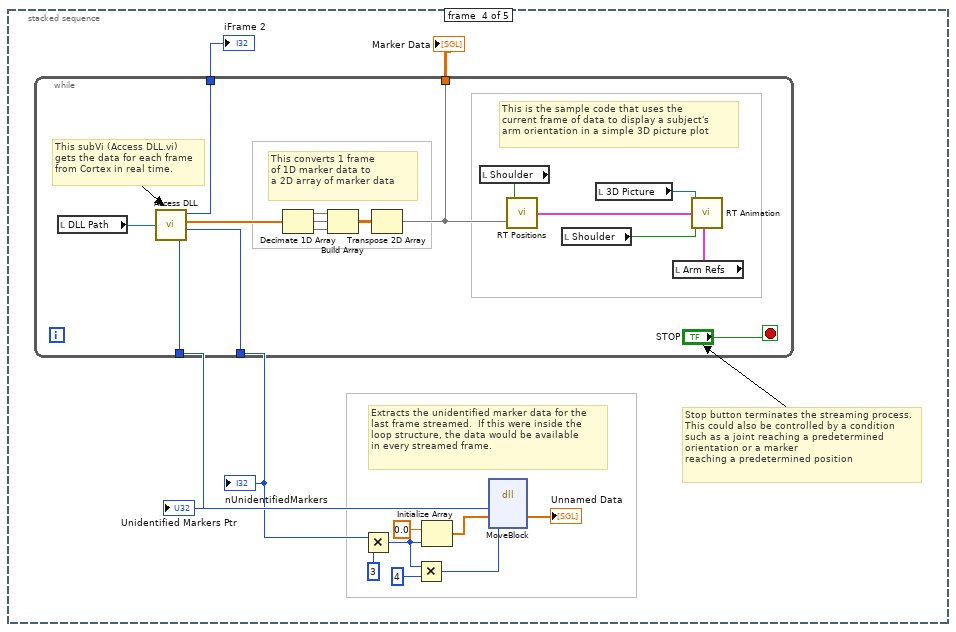
[diagram p4: hidden frame]
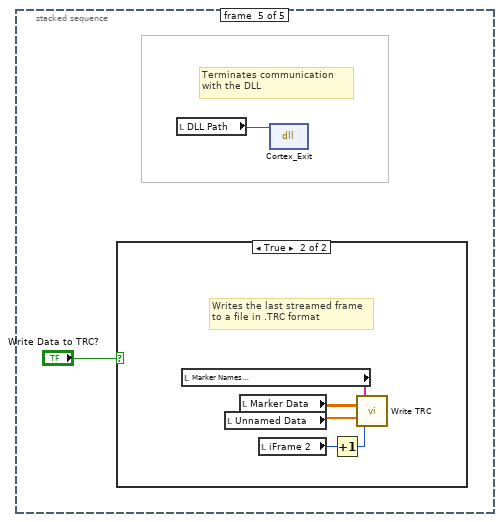
[diagram p5: hidden frame]
diagram:
  n1 = stacked-sequence {
    frame #0 {
      w2 = 0.0
      # "This code sets the parameters for displaying the 3D picture in this example.  It is not part of the SDK code that communicates with Cortex.\nWhen modifying this code for their own purpose, users not creating a picture file (3D animated display) will delete this frame."
      n2 = call <vilib>:"Setup Window.vi"("Camera Controller"=enum16{"None", "Spherical", "Flying"}."Spherical", "Window State"=T4."Open") -> ("New Window Refnum"=w18:refnum<vi>)  [unwired: 8 in, 1 out]
      n3 = invoke class="SceneWindow" method="Setup Camera"(reference=w18, "Camera Position"=T5 {"X"=12.0, "Y"=0.0, "Z"=0.0}, "Target"=T5 {"X"=0.0, "Y"=1.0, "Z"=0.0} ("Camera Position"), "Up Direction"=T5 {"X"=0.0, "Y"=0.0, "Z"=1.0} ("Camera Position")) -> (reference out=w17:refnum<vi>)  [unwired: 2 in, 5 out]
      n4 = Array To Cluster(array=dbl[] [0.0, 0.0, 0.0] ("Shoulder Axis")) -> (cluster=w5:T7)
      n5 = Bundle(w2, "Shoulder Axis"=w5, w2, "Shoulder Axis"=w5, "Humerus Coord Sys"=T3 [], "Shoulder Axis"=w5) -> (w1:T8)  [unwired: 1 in]
      n6 = local read "Shoulder"() -> (w10:bool)
      n7 = property class="SceneWindow"(reference=w17, "WinBounds"=T6 {"Left"=590, "Top"=100, "Right"=1190, "Bottom"=700} ("Window Bounds"), "AutoProjection"=enum16{"None", "Perspective", "Orthographic"}."None" ("Automatic Projection Mode"), "State"=T4."Open" ("Window State")) -> (reference out=w9:refnum<vi>)  [unwired: 1 in, 1 out]
      "SceneWindow" <- w9
      n8 = call "Create Animation.vi"("L/R"=w10, "Target Values"=w1) -> ("Arm Refs"=→"Arm Refs":T2, "Scene Out"=w8:refnum<vi>)  [unwired: 1 in]
      n9 = property class="SceneWindow"(reference=w9, "Scene"=w8) -> (reference out=→"3D Picture":refnum<vi>)  [unwired: 1 in, 1 out]
    }
    frame #1 {
      # "Initialize the connection between \nthe Cortex machine (Host) and the \nmachine processing the real-time\ndata stream (Local).  This is part of the \nLabView-SDK interface."
      n10 = dll-call lib="?" fn="Cortex_Initialize"(path in="DLL Path", "Local_IP"="Local IP", "Eva_IP"="Host IP") -> ()  [unwired: 5 in, 2 out]
    }
    frame #2 {
      w60 = 1 ("dimension size")
      # "Max marker name length is\n64 characters, so the total number\nof bytes to be read  is nMarkers * 64"
      # "Convert the  marker\nname data from U8\ndata type to character"
      # "Use the pointer to\nextract the  marker\nname data"
      # "Use the handle to\nextract the pointer\nto the marker names"
      # "Extract the number of sBodyDef\nstructures defined by nBodyDefs"
      # "sBodyDefs contains 805 32-bit words,\nand each 32 bit word is 4 bytes, for a total of\n805 * 4 bytes."
      # "Retrieves  sBodyDefs  data\nusing pointer address"
      # "Retrieves pointer to sBodyDefs \nfrom Cortex_SDK.dll"
      # "This creates the structure for sBodyDefs as documented in the Cortex.h file."
      # "Extract the number of markers\n from the first sBodyDef"
      n11 = Unbundle By Name("sBodyDefs") -> ("nBodyDefs"=w30:i32, "sBodyDef"=w27:T9, "nAnalogChannels"=w32:i32, "szAnalogChannelNames"=w33:u32, "nForcePlates"=w34:i32, "AllocatedSpace"=w39:u32)
      n12 = for {
        N: 100 -> [_]
        tunnel: w27 -> [w77]
        tunnel: [w77] -> w29 mode=indexing
      }
      n13 = local read "DLL Path"() -> (w24:path)
      n14 = Array To Cluster(array=w29) -> (cluster=w31:T10)
      n15 = Bundle("nBodyDefs"=w30, w31, "nAnalogChannels"=w32, "szAnalogChannelNames"=w33, "nForcePlates"=w34, "AllocatedSpace"=w39) -> (w41:T11)  [unwired: 1 in]
      n16 = dll-call lib="?" fn="Cortex_GetBodyDefs"(path in=w24) -> ("return type"=w25:u32)  [unwired: 2 in, 2 out]
      n17 = Multiply(x=805, y=4) -> (x*y=w44:i32)
      n18 = dll-call lib="LabVIEW" fn="MoveBlock"("Pointer"=w25, "Array"=w41, "Length"=w44) -> ("Array"=w40:T11)  [unwired: 6 in, 2 out]
      n19 = Unbundle(w40) -> ("nBodyDefs"=w64:i32, w35:T10)  [unwired: 4 out]
      n20 = Cluster To Array(cluster=w35) -> (array=w36:T12)
      n21 = Array Subset(array=w36, index=0, length=w64) -> (w38:T12)
      n22 = for {
        tunnel: w38 -> [w75] mode=indexing
        tunnel: [w74] -> w56 mode=indexing
        tunnel: [w76] -> w62 mode=indexing
        n23 = Unbundle(w75) -> ("nMarkers"=w76:i32, "szMarkerNames"=w74:u32)  [unwired: 4 out]
      }
      "nMarkers" <- w62
      "szMarkerNames" <- w56
      n24 = Multiply(x=w60, y=4) -> (x*y=w50:i32)
      n25 = Index Array(array=w56, index=0) -> (element=w57:u32)
      n26 = Initialize Array(u32 0 ("element"), w60) -> (w61:u32[])
      n27 = Index Array(array=w62, index=0) -> (element=w65:i32)
      "Number of Markers\nfor first BodyDef" <- w65
      n28 = dll-call lib="LabVIEW" fn="MoveBlock"("Pointer"=w57, "Array"=w61, "Length"=w50) -> ("Array"=w51:u32[])  [unwired: 6 in, 2 out]
      n29 = Multiply(x=u32 64 ("y"), y=w65) -> (x*y=w48:u32)
      n30 = Index Array(array=w51, index=0) -> (element=w53:u32)
      n31 = Initialize Array(u8 0 ("element"), w48) -> (w46:u8[])
      n32 = dll-call lib="LabVIEW" fn="MoveBlock"("Pointer"=w53, "Array"=w46, "Length"=w48) -> ("Array"=w49:u8[])  [unwired: 6 in, 2 out]
      n33 = for {
        N: w65 -> [_]
        shift-right: [w66] -> _
        shift-left: w49 -> [w72]
        tunnel: [w70] -> w58 mode=indexing
        n34 = Search 1D Array(1D array=w72, element=u8 0) -> (index of element=w73:i32)  [unwired: 1 in]
        n35 = Split 1D Array(array=w72, index=w73) -> (first subarray=w71:u8[], second subarray=w68:u8[])
        n36 = Byte Array To String(unsigned byte array=w71) -> (string=w70:string)
        n37 = Array Subset(array=w68, index=1) -> (w66:u8[])  [unwired: 1 in]
      }
      "Marker Names\nfor first BodyDef" <- w58
    }
    frame #3 {
      # "Stop button terminates the streaming process.  This could also be controlled by a condition such as a joint reaching a predetermined orientation or a marker \nreaching a predetermined position"
      # "Extracts the unidentified marker data for the \nlast frame streamed.  If this were inside the \nloop structure, the data would be available\nin every streamed frame."
      n38 = while {
        tunnel: [w94] -> w81
        tunnel: [w93] -> w82
        tunnel: [w90] -> w79
        tunnel: [w89] -> w78
        stop <- "STOP" stop-if-true
        # "This is the sample code that uses the \ncurrent frame of data to display a subject's\narm orientation in a simple 3D picture plot"
        # "This converts 1 frame\nof 1D marker data to\na 2D array of marker data"
        # "This subVi (Access DLL.vi) \ngets the data for each frame\nfrom Cortex in real time."
        n39 = local read "DLL Path"() -> (w104:path)
        n40 = call "Access DLL.vi"("DLL Path"=w104) -> ("iFrame"=w89:i32, "Marker Data"=w96:sgl[], "nUnidentifiedMarkers"=w94:i32, "Unidentified Markers Ptr"=w93:u32)
        n41 = Decimate 1D Array(w96) -> (w103:sgl[], w102:sgl[], w101:sgl[])
        n42 = Build Array(w103, w102, w101) -> (w100:sgl[][])
        n43 = Transpose 2D Array(2D array=w100) -> (transposed array=w90:sgl[][])
        n44 = local read "Shoulder"() -> (w97:bool)
        n45 = call "RT Positions.vi"("Coordinates"=w90, "L/R"=w97) -> ("Cluster"=w95:T13)
        n46 = local read "Shoulder"() -> (w92:bool)
        n47 = local read "3D Picture"() -> (w99:refnum<vi>)
        n48 = local read "Arm Refs"() -> (w98:T2)
        n49 = call "RT Animation.vi"("3D Picture"=w99, "RT Position"=w95, "Left/Right"=w92, "Arm Refs"=w98) -> ()  [unwired: 3 in]
      }
      "Unidentified Markers Ptr" <- w82
      "nUnidentifiedMarkers" <- w81
      "Marker Data" <- w79
      "iFrame 2" <- w78
      n50 = Multiply(x=w81, y=3) -> (x*y=w86:i32)
      n51 = Multiply(x=w86, y=4) -> (x*y=w88:i32)
      n52 = Initialize Array(sgl 0.0 ("index"), w86) -> (w85:sgl[])
      n53 = dll-call lib="LabVIEW" fn="MoveBlock"("Pointer"=w82, "array"=w85, "Length"=w88) -> ("array"=→"Unnamed Data":sgl[])  [unwired: 6 in, 2 out]
    }
    frame #4 {
      # "Terminates communication \nwith the DLL"
      n54 = case shown="True" "Write Data to TRC?" {
        frame False {
        }
        frame True {
          # "Writes the last streamed frame\nto a file in .TRC format"
          n55 = local read "Marker Names\nfor first BodyDef"() -> (w107:string[])
          n56 = local read "Unnamed Data"() -> (w108:sgl[])
          n57 = local read "Marker Data"() -> (w109:sgl[][])
          n58 = local read "iFrame 2"() -> (w111:i32)
          n59 = Increment(x=w111) -> (x+1=w110:i32)
          n60 = call "Write TRC.vi"("Frame"=w110, "Unidentified Data"=w108, "Marker Data"=w109, "Markers"=w107) -> ()  [unwired: 1 in]
        }
      }
      n61 = local read "DLL Path"() -> (w105:path)
      n62 = dll-call lib="?" fn="Cortex_Exit"(path in=w105) -> ()  [unwired: 3 in, 2 out]
    }
  }
